vi "XY Graph Get Plots Metadata.vi"(8 "Error In":errorcluster, 11 "XYGraph Ref":T1) -> (0 "Error Out":errorcluster, 1 "Plots Metadata Found?":bool, 2 "Plots Metadata":variant[](array[variant]), 3 "XYGraph Ref (dup)":T1)   [LabVIEW 2019, in "XY Graph Add-Ons.lvlib"]
uses:
  XY Graph Add-Ons.lvlib
  XY Graph Refnum.ctl
  XY Graph Property Tag List.ctl
  <vilib>/UserTags/UserTags.lvlib
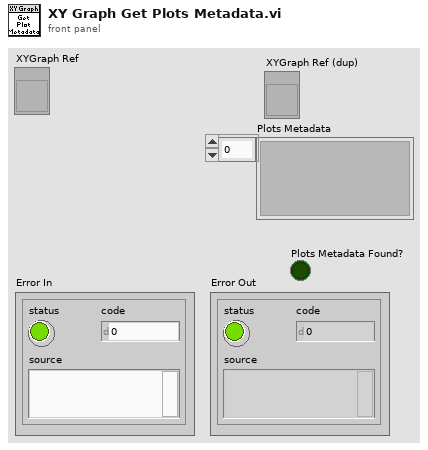
[diagram p1: front panel]
types:
  T1 = typedef "XY Graph Add-Ons.lvlib/XY Graph Refnum.ctl" = refnum<vi>
  T2 = typedef "XY Graph Add-Ons.lvlib/XY Graph Property Tag List.ctl" = enum16{"Max Legend Size", "Preserved Plots", "XScales.GridColors", "YScales.GridColors", "TipStrip String", "TipStrip Visible", "Tool Panels Visibility", "Plots Metadata"}
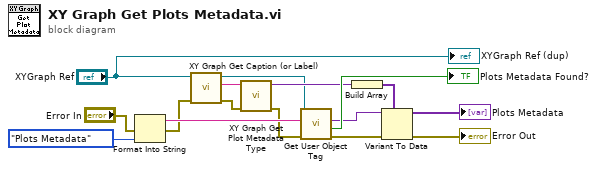
[diagram p0: block diagram]
diagram:
  n1 = Format Into String(error in="Error In", XY_Graph_Property_Tag_List."Plots Metadata" ("XY Graph Property Tag")) -> (resulting string=w14:string, error out=w4:errorcluster)  [unwired: 2 in]
  n2 = call "XY Graph Get Caption (or Label).vi"("error in (no error)"=w4, "XYGraph in"="XYGraph Ref") -> ("error out"=w3:errorcluster, "Caption (or Label) Text"=w10:string, "XYGraph out"=w6:T1)  [unwired: 7 in]
  n3 = call "XY Graph Get Plot Metadata Type.vi"("Error In"=w3, "Graph Label"=w10) -> ("Error Out"=w8:errorcluster, "Plot Metadata Type"=w9:variant)  [unwired: 7 in, 1 out]
  n4 = call <vilib>:"Get User Object Tag.vi"("error in (no error)"=w8, "Tag Name"=w14, "Generic Refnum"=w6) -> ("error out"=w12:errorcluster, "Was Tag Found?"=→"Plots Metadata Found?":bool, "Value"=w13:variant)  [unwired: 5 in, 1 out]
  n5 = Build Array(w9) -> (w7:variant[])
  n6 = Variant To Data(error in=w12, type=w7, Variant=w13) -> (data=→"Plots Metadata":variant[], error out=→"Error Out":errorcluster)
  "XYGraph Ref (dup)" <- "XYGraph Ref"
